vi "Frame.vi"(8 "error in (no error)":errorcluster, 11 "Node Ptr":T4 format="%.0x") -> (0 "error out":errorcluster)   [LabVIEW 2020, in "AIM ARINC 664 System Explorer.lvlib" / "Implementation.lvlib"]
uses:
  Implementation.lvlib
  <vilib>/NI VeriStand/Custom Device API/Custom Device Item Ref.ctl
  Import/_typedefs/frame_tx_generic_seqNumberInit.ctl
  Import/_typedefs/frame_tx_generic_seqNumberOffset.ctl
  Scripting/Constants.vi
  <vilib>/NI VeriStand/Custom Device API/Get Item Property (String).vi
  <vilib>/NI VeriStand/Custom Device API/Custom Device API.lvlib
  Frame Configuration/FrameEditor.lvlib
  Scripting/AIM ARINC 664 Scripting.lvlib
  <instrlib>/AIM GmbH/_AIM 664/AIM664LV.lvlib
  <vilib>/Utility/Data Type/NI_Data Type.lvlib
  Import/AIM ARINC 664 Import.lvlib
panel:
  in  "SHDocVw.IWebBrowser":refnum<k7>(container)
  in  "Specific Header":cluster{"Section Name":string}={"Section Name"="Specific Page Settings"}
  in  "General Header":cluster{"Section Name":string}={"Section Name"="General Page Settings"}
  in  "Description":string
  in  "Name":string
  in  "Property List":i32(listbox)
  in  "Frame header":T3 {"FrameStartMode" items=["FDX_TX_FRAME_START_IFG", "FDX_TX_FRAME_START_PGWT", "FDX_TX_FRAME_START_TRG", "FDX_TX_FRAME_START_TRG_D"]; "NetSelect" items=["FDX_TX_FRAME_DLY_A", "FDX_TX_FRAME_DLY_B", "FDX_TX_FRAME_BOTH", "FDX_TX_FRAME_ONLY_A", "FDX_TX_FRAME_ONLY_B"]; "PayloadBufferMode" items=["FDX_TX_FRAME_PBM_STD", "FDX_TX_FRAME_PBM_MAC", "FDX_TX_FRAME_PBM_UDP", "FDX_TX_FRAME_PBM_FULL"]; "PayloadGenerationMode" items=["FDX_TX_FRAME_PGM_USER", "FDX_TX_FRAME_PGM_IP_PART", "FDX_TX_FRAME_PGM_IP_PART_TT", "FDX_TX_FRAME_PGM_IP_FULL", "FDX_TX_FRAME_PGM_IP_FULL_TT"]; "PhysErrorInjection" items=["FDX_TX_FRAME_ERR_OFF", "FDX_TX_FRAME_ERR_CRC", "FDX_TX_FRAME_ERR_ALI", "FDX_TX_FRAME_ERR_PRE", "FDX_TX_FRAME_ERR_PHY"]; "SequenceNumberInit" items=["FDX_TX_FRAME_SEQ_INIT_AUTO"=65535, "FDX_TX_FRAME_SEQ_OFF"=65533]; "SequenceNumberOffset" items=["FDX_TX_FRAME_SEQ_OFFS_AUTO"=65535]}
  in  "Properties":string(tree)
  out "Frame Data":string[][](table)
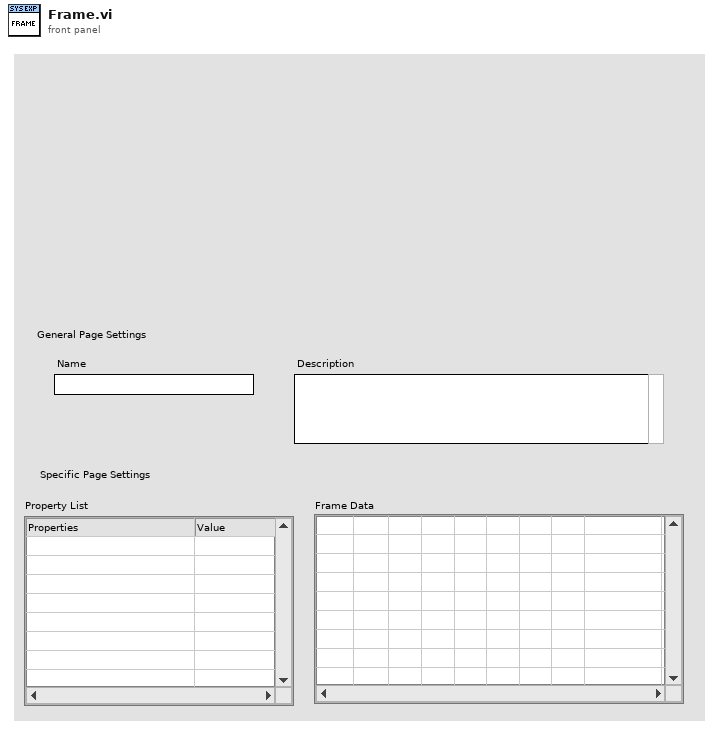
[diagram p1: front panel]
types:
  T1 = typedef "AIM ARINC 664 Import.lvlib/frame_tx_generic_seqNumberInit.ctl" = i32
  T2 = typedef "AIM ARINC 664 Import.lvlib/frame_tx_generic_seqNumberOffset.ctl" = i32
  T3 = cluster{"FrameStartMode":i32, "InterFrameGap":i32, "PacketGroupWaitTime":i32, "NetSelect":i32, "PayloadBufferMode":i32, "PayloadGenerationMode":i32, "PhysErrorInjection":i32, "PreambleCount":i32, "SequenceNumberInit":T1, "SequenceNumberOffset":T2, "Skew":i32}
  T4 = typedef "Custom Device API.lvlib/Custom Device Item Ref.ctl" = u64
  T5 = typedef "Custom Device API.lvlib/Custom Device Item Info.ctl" = cluster{"Name":string, "Is Channel":bool, "GUID":string, "Is Waveform":bool}
  T6 = cluster{"Left Cell String":string, "Child Text":string[], "Child Tag":string, "Item Indent":i32, "Child Only?":bool, "Glyph Index":i32}
  T7 = typedef "Custom Device API.lvlib/Custom Device Commands.ctl" = enum16{"Default", "Item renamed", "Shutdown", "Dynamic button pressed"}
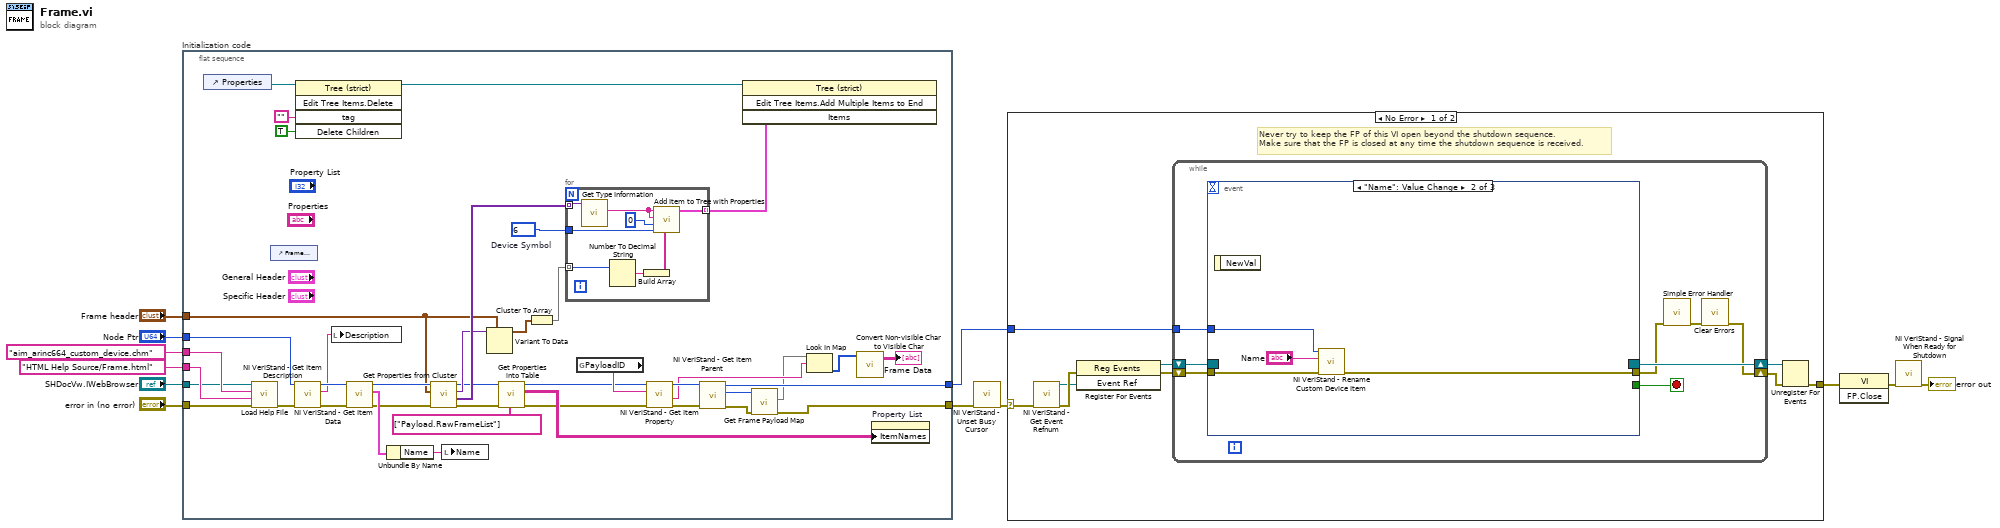
[diagram p0: block diagram]
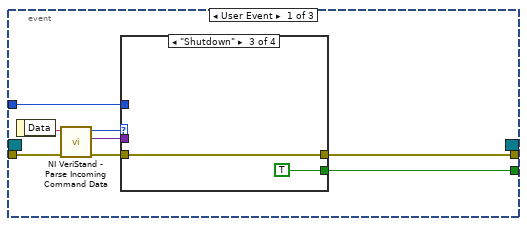
[diagram p2: hidden frame]
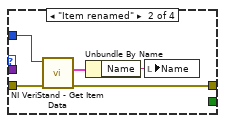
[diagram p4: hidden frame]
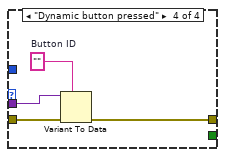
[diagram p5: hidden frame]
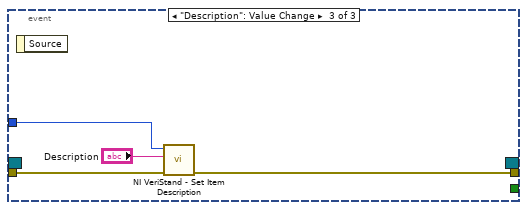
[diagram p6: hidden frame]
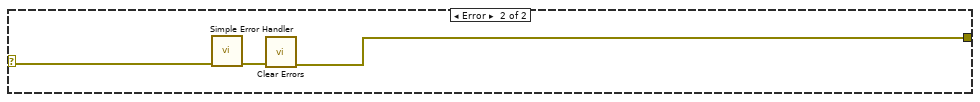
[diagram p7: hidden frame]
diagram:
  n1 = flat-sequence "Initialization code" {
    tunnel: "error in (no error)" -> [w47]
    tunnel: "Node Ptr" -> [w50]
    tunnel: [w14] -> w8
    tunnel: [w19] -> w5
    tunnel: "SHDocVw.IWebBrowser" -> [w43]
    tunnel: "HTML Help Source/Frame.html" ("CD_CHM_Section") -> [w45]
    tunnel: "aim_arinc664_custom_device.chm" ("CD_CHM_FileName") -> [w44]
    tunnel: "Frame header" -> [w32]
    frame #0 {
      w33 = 6  # Device Symbol
      n2 = control-ref of="Properties"() -> (w26:refnum<vi>)
      n3 = call "Load Help File.vi"("error in (no error)"=w47, "HTML File to Load"=w45, "Main CHM File"=w44, "Browser"=w43) -> ("error out"=w46:errorcluster)  [unwired: 6 in, 1 out]
      n4 = control-ref of="Frame header"() -> ()  [unwired: 1 out]
      n5 = call <vilib>:"NI VeriStand - Get Item Description.vi"("error in (no error)"=w46, "Item Ref in"=w50) -> ("error out"=w52:errorcluster, "Description"=w48:string, "Item Ref out"=w53:T4)  [unwired: 7 out]
      n6 = invoke on="Invoke Node" class="Tree (strict)" method="Edit Tree Items.Delete"(reference=w26, "tag"="", "Delete Children"=TRUE ("Delete Children?")) -> (reference out=w23:refnum<vi>)  [unwired: 2 in, 4 out]
      n7 = local write "Description"(w48) -> ()
      n8 = call <vilib>:"NI VeriStand - Get Item Data.vi"("error in (no error)"=w52, "Item Ref in"=w53) -> ("error out"=w39:errorcluster, "Item Info"=w51:T5, "Item Ref out"=w40:T4)  [unwired: 7 out]
      n9 = Unbundle By Name(w51) -> ("Name"=w49:string)
      n10 = call "Get Properties from Cluster.vi"("error in"=w39, "Variant Cluster"=w32, "custom device ref in"=w40) -> ("error out"=w28:errorcluster, "Array"=w38:variant[], "data"=w36:variant, "custom device ref out"=w30:T4)  [unwired: 5 in]
      n11 = local write "Name"(w49) -> ()
      n12 = Variant To Data(type=w32, Variant=w36) -> (data=w35:T3)  [unwired: 1 in, 1 out]
      n13 = call "Get Properties into Table.vi"("Blacklisted properites"=string[] ["Payload.RawFrameList"], "error in"=w28, "Item Ref in"=w30) -> ("error out"=w27:errorcluster, "Property Names"=w31:string[][], "Item Ref out"=w29:T4)  [unwired: 6 in]
      n14 = Cluster To Array(cluster=w35) -> (array=w34:T2[])
      n15 = for {
        tunnel: w38 -> [w61] mode=indexing
        tunnel: [w59] -> w37 mode=indexing
        tunnel: w34 -> [w58] mode=indexing
        tunnel: w33 -> [w54]
        n16 = call <vilib>:"Get Type Information.vi"("variant"=w61) -> ("name"=w60:string)  [unwired: 6 in, 4 out]
        n17 = Number To Decimal String(number=w58) -> (decimal integer string=w56:string)  [unwired: 1 in]
        n18 = Build Array(w56) -> (w55:string[])
        n19 = call <instrlib>:"Add Item to Tree with Properties.vi"("Child Text"=w55, "Glyph Index"=w54, "Item indent"=0, "Child Tag"=w60, "Left Cell String"=w60) -> ("Item"=w59:T6)  [unwired: 6 in]
      }
      n20 = global read "Constants.vi" "PayloadID"() -> (w41:string)
      n21 = call-poly <vilib>:"NI VeriStand - Get Item Property.vi"("error in (no error)"=w27, "Property Name"=w41, "Item Ref in"=w29) -> ("error out"=w20:errorcluster, "Value"=w18:string, "Item Ref out"=w21:T4)  [unwired: 5 in, 1 out]
      n22 = call <vilib>:"NI VeriStand - Get Item Parent.vi"("error in (no error)"=w20, "Item Ref in"=w21) -> ("error out"=w15:errorcluster, "Parent Ref"=w16:T4, "Item Ref out"=w19:T4)  [unwired: 6 in, 1 out]
      n23 = invoke on="Invoke Node" class="Tree (strict)" method="Edit Tree Items.Add Multiple Items to End"(reference=w23, "Items"=w37) -> ()  [unwired: 2 in, 4 out]
      n24 = call "Get Frame Payload Map.vi"("error in"=w15, "custom device ref in"=w16) -> ("error out"=w14:errorcluster, "Payload Map"=w13:map{string, u8[]})  [unwired: 7 in, 1 out]
      n25 = Look In Map(map=w13, key=w18) -> (value=w17:u8[])  [unwired: 1 in, 1 out]
      n26 = call "Convert Non-visible Char to Visible Char.vi"("data"=w17) -> ("data table"=→"Frame Data":string[][])  [unwired: 8 in, 2 out]
      n27 = property on="Property List" class="MCListbox (strict)"("ItemNames"=w31) -> ()  [unwired: 2 in, 2 out]
    }
  }
  n28 = call <vilib>:"NI VeriStand - Unset Busy Cursor.vi"("error in (no error)"=w8) -> ("error out"=w7:errorcluster)  [unwired: 10 out]
  n29 = case shown="No Error" w7 {
    selector: w7 -> [w62 w109]
    tunnel: [w67 w107] -> w12
    tunnel: w5 -> [w63 _]
    frame No Error {
      # "Never try to keep the FP of this VI open beyond the shutdown sequence.\nMake sure that the FP is closed at any time the shutdown sequence is received."
      n30 = call <vilib>:"NI VeriStand - Get Event Refnum.vi"("error in (no error)"=w62) -> ("error out"=w70:errorcluster, "Event Ref"=w66:refnum<user-event>)  [unwired: 9 out]
      n31 = register-events(error in=w70, w66) -> (reference out=w64:refnum<event-registration>, error out=w65:errorcluster)  [unwired: 1 in]
      n32 = while {
        tunnel: w63 -> [w74]
        shift-right: [w71] -> w68
        shift-left: w65 -> [w77]
        shift-right: [w78] -> w69
        shift-left: w64 -> [w76]
        stop <- w75 stop-if-true
        n33 = event shown="[1] \"Name\": Value Change" {
          selector: w76 -> [_ _ _]
          dyn-events: [_ _ _] -> w78
          timeout: _ -> [_ _ _]
          tunnel: w77 -> [w86 w102 w105]
          tunnel: [w82 _ _] -> w75
          tunnel: [w81 w101 w104] -> w73
          tunnel: w74 -> [w80 w100 w106]
          event User Event {
            n34 = event-data() -> ("Data"=w85:string)  [unwired: 1 out]
            n35 = call <vilib>:"NI VeriStand - Parse Incoming Command Data.vi"("error in (no error)"=w86, "Incoming data"=w85) -> ("error out"=w84:errorcluster, "Outgoing data"=w79:variant, "Action"=w83:T7)  [unwired: 7 out]
            n36 = case shown="\"Shutdown\"" w83 {
              tunnel: w84 -> [w87 w92 w93 w98]
              tunnel: [_ _ TRUE _] -> w82
              tunnel: [w87 w89 w93 w95] -> w81
              tunnel: w80 -> [_ w91 _ _]
              tunnel: w79 -> [_ _ _ w97]
              frame "Default", Default {
              }
              frame "Item renamed" {
                n37 = call <vilib>:"NI VeriStand - Get Item Data.vi"("error in (no error)"=w92, "Item Ref in"=w91) -> ("error out"=w89:errorcluster, "Item Info"=w90:T5)  [unwired: 8 out]
                n38 = Unbundle By Name(w90) -> ("Name"=w88:string)
                n39 = local write "Name"(w88) -> ()
              }
              frame "Shutdown" {
              }
              frame "Dynamic button pressed" {
                w96 = ""  # Button ID
                n40 = Variant To Data(error in=w98, type=w96, Variant=w97) -> (error out=w95:errorcluster)  [unwired: 1 out]
              }
            }
          }
          event "Name": Value Change {
            n41 = event-data() -> ()  [unwired: 2 out]
            n42 = call <vilib>:"NI VeriStand - Rename Custom Device Item.vi"("error in (no error)"=w102, "New Name"="Name", "Item Ref in"=w100) -> ("error out"=w101:errorcluster)  [unwired: 1 in, 7 out]
          }
          event "Description": Value Change {
            n43 = event-data() -> ()  [unwired: 2 out]
            n44 = call <vilib>:"NI VeriStand - Set Item Description.vi"("error in (no error)"=w105, "Description"="Description", "Item Ref in"=w106) -> ("error out"=w104:errorcluster)  [unwired: 8 out]
          }
        }
        n45 = call <vilib>:"Simple Error Handler.vi"("error in (no error)"=w73) -> ("error out"=w72:errorcluster)  [unwired: 1 in, 7 out]
        n46 = call <vilib>:"Clear Errors.vi"("error in (no error)"=w72) -> ("error out"=w71:errorcluster)  [unwired: 1 in, 5 out]
      }
      n47 = Unregister For Events(event registration refnum=w69, error in=w68) -> (error out=w67:errorcluster)
    }
    frame Error {
      n48 = call <vilib>:"Simple Error Handler.vi"("error in (no error)"=w109) -> ("error out"=w108:errorcluster)  [unwired: 1 in, 7 out]
      n49 = call <vilib>:"Clear Errors.vi"("error in (no error)"=w108) -> ("error out"=w107:errorcluster)  [unwired: 1 in, 5 out]
    }
  }
  n50 = invoke class="VI" method="FP.Close"(error in=w12) -> (error out=w11:errorcluster)  [unwired: 2 in, 2 out]
  n51 = call <vilib>:"NI VeriStand - Signal When Ready for Shutdown.vi"("error in (no error)"=w11) -> ("error out"=→"error out":errorcluster)  [unwired: 10 out]
